vi "Data Viewer.vi"(8 "error in":errorcluster) -> (0 "error out":errorcluster)   [LabVIEW 2019, in "Report Viewer.lvlib" / "Report Viewer.lvclass"]
uses:
  Library/Report Viewer.lvclass
  Library/Report Viewer.lvclass/Report Viewer.ctl
  Accessors/Write Filename_ref.vi
  Accessors/GUI/Write Tree Refnum.vi
  Accessors/GUI/Write Graph_Ref.vi
  Accessors/GUI/Write Properties_Ref.vi
  Accessors/GUI/Write Values_Ref.vi
  Accessors/GUI/Write VI Refnum.vi
  Accessors/GUI/Write Save Data Button.vi
  Private/Tree/Clear Tree.vi
panel:
  in  "File contents":string[](tree)
  in  "Stop":bool
  out "File Name":string
  in  "Settings":bool
  in  "Open TDMS":bool
  in  "Save Graph":bool
  in  "Export Table":bool
  in  "Tab Control":T1(tab)
  in  "Properties Table":i32(listbox)
  in  "Values Table":i32(listbox)
  out "Waveform Graph":waveform(dbl)[](graph)
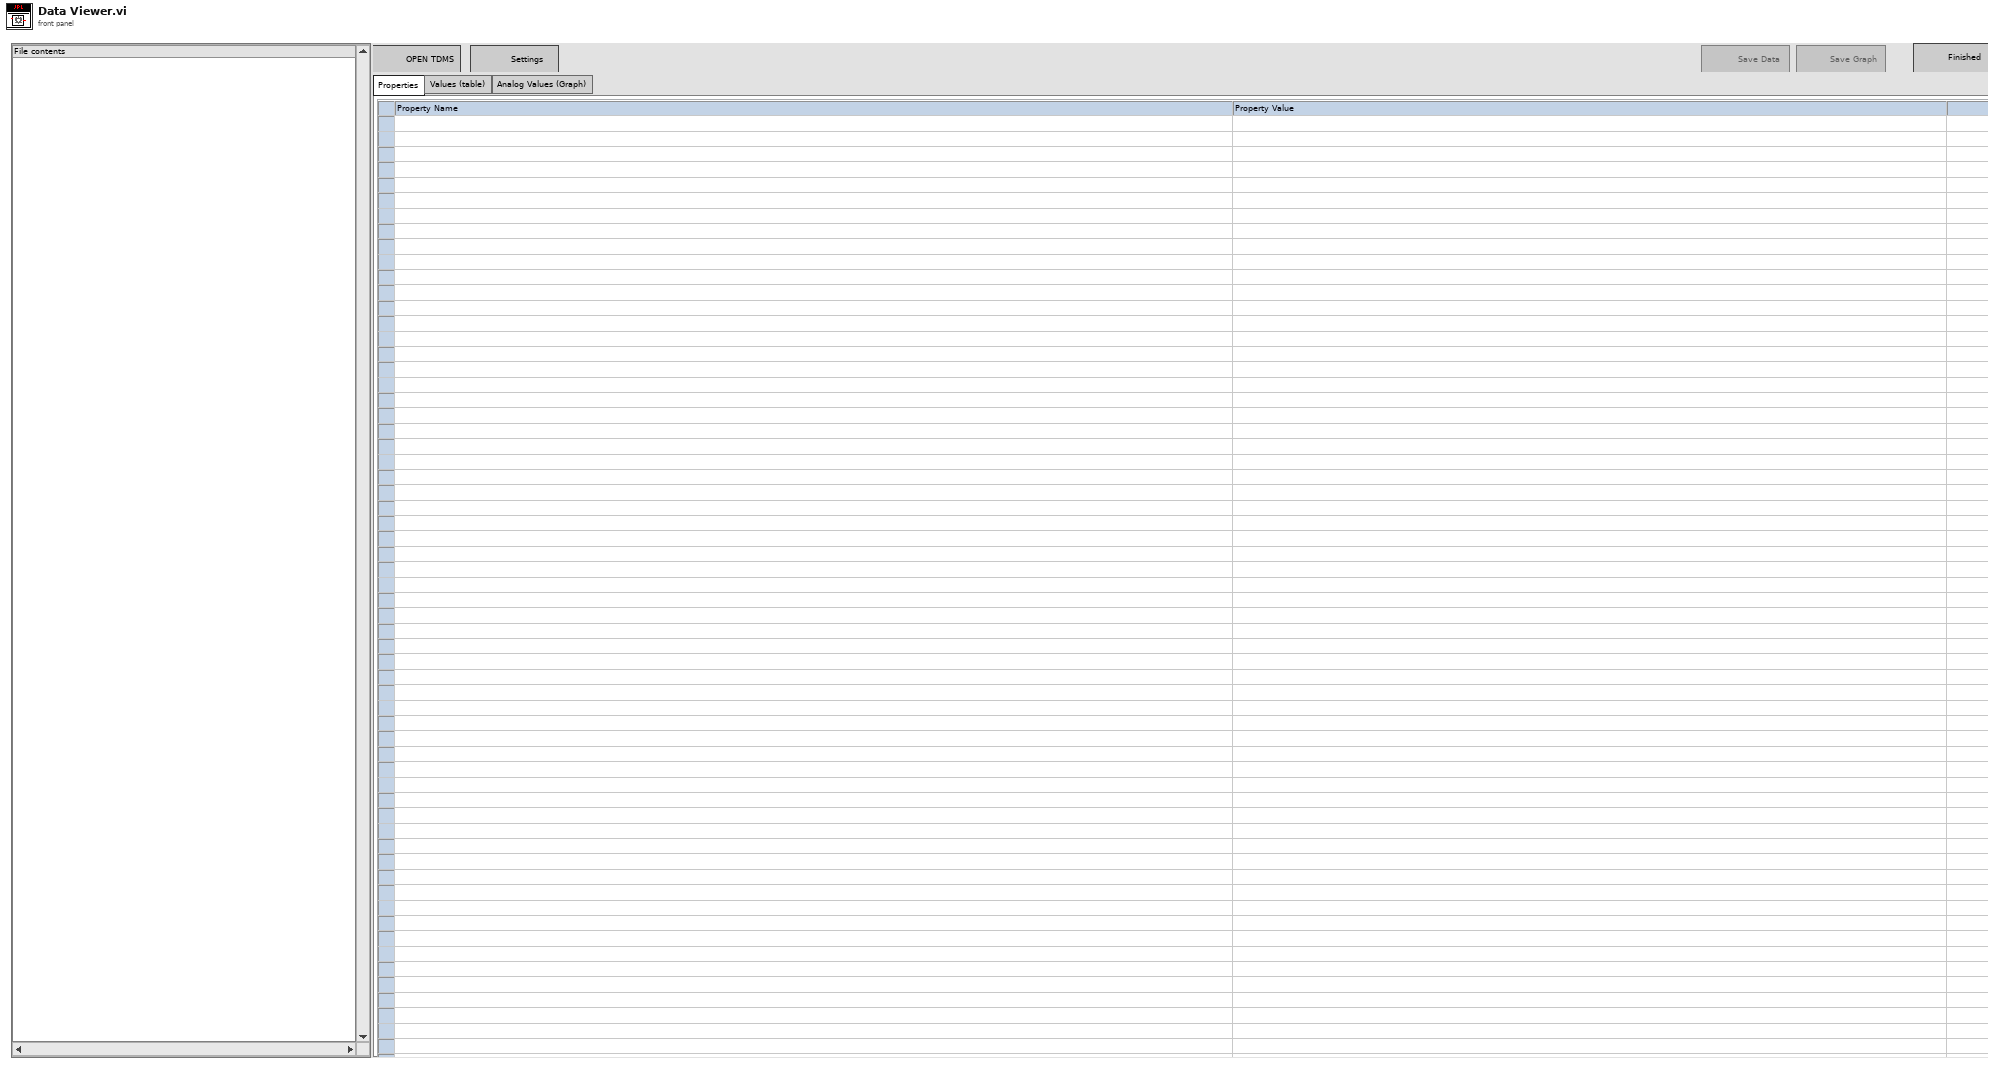
[diagram p1: front panel]
types:
  T1 = enum32{"Properties", "Values (table)", "Analog Values (Graph)"}
  T2 = typedef "LVBoundsTypeDef.ctl" = cluster{"Width":u32, "Height":u32}
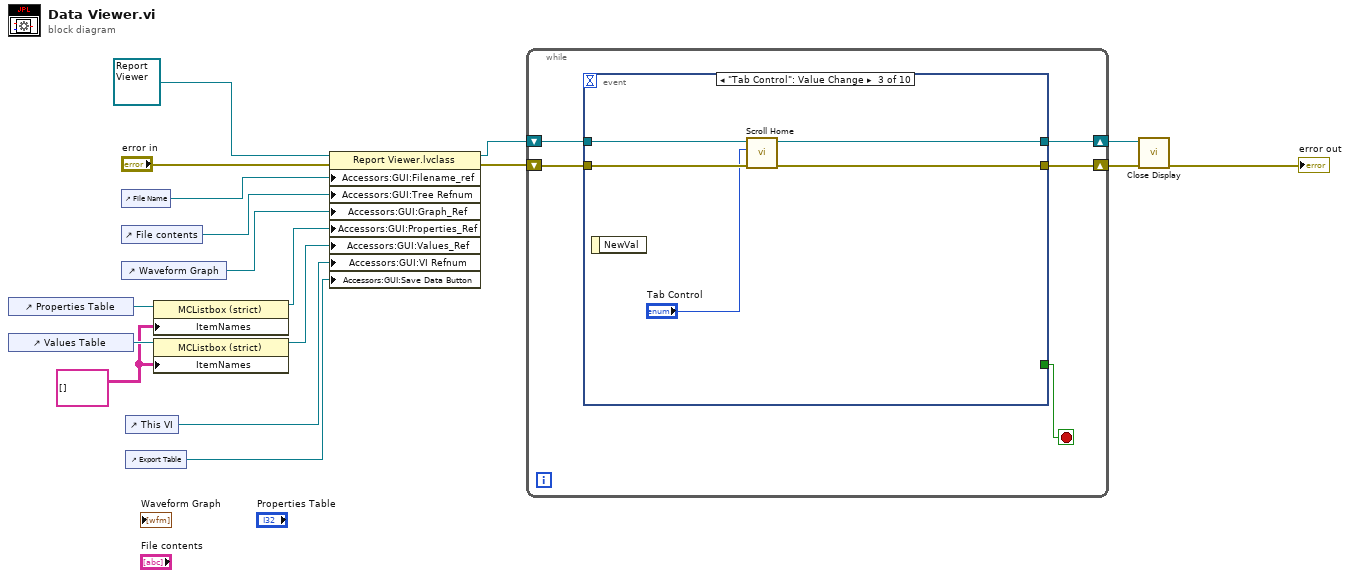
[diagram p0: block diagram]
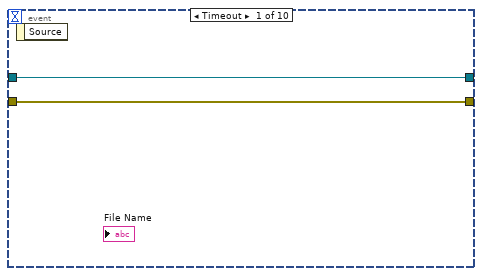
[diagram p2: hidden frame]
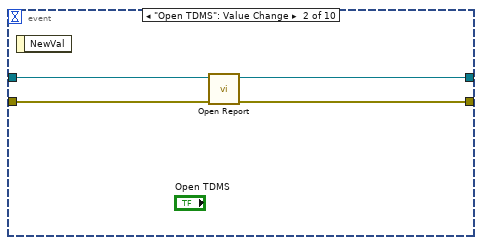
[diagram p3: hidden frame]
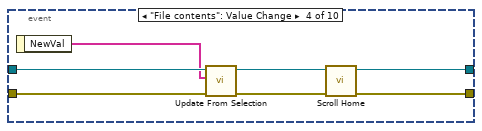
[diagram p4: hidden frame]
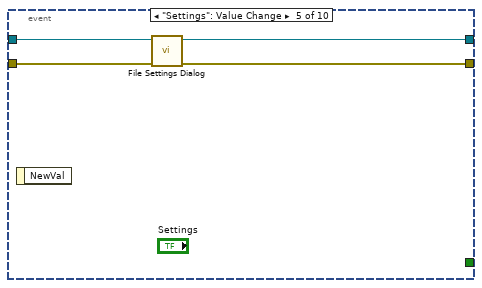
[diagram p5: hidden frame]
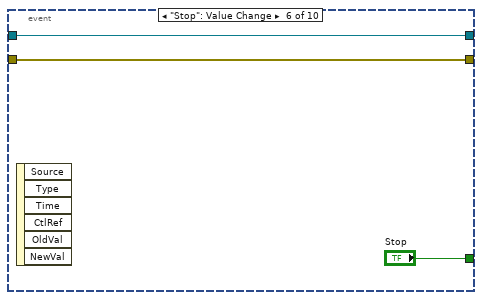
[diagram p6: hidden frame]
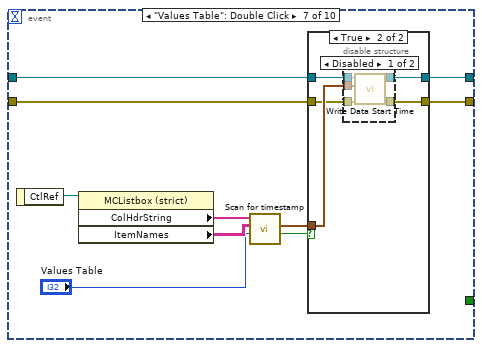
[diagram p7: hidden frame]
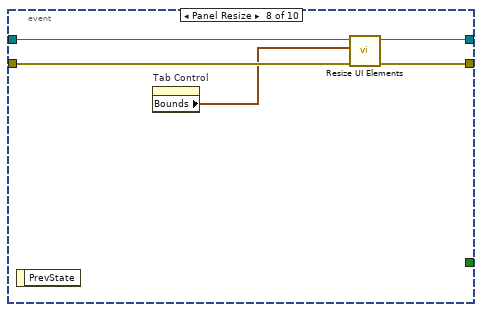
[diagram p10: hidden frame]
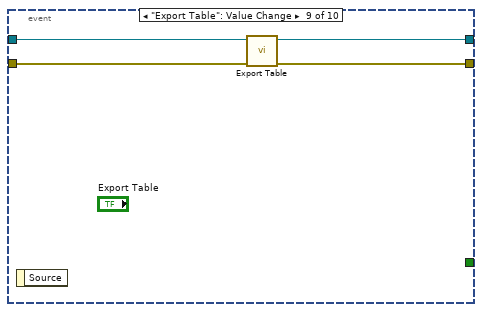
[diagram p11: hidden frame]
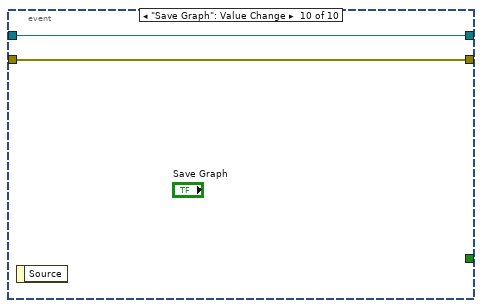
[diagram p12: hidden frame]
diagram:
  w5 = string[][] [] ("Item Names")
  n1 = control-ref of="Properties Table"() -> (w9:refnum<vi>)
  n2 = control-ref of="Values Table"() -> (w7:refnum<vi>)
  n3 = control-ref of="File Name"() -> (w14:refnum<vi>)
  n4 = control-ref of="File contents"() -> (w13:refnum<vi>)
  n5 = control-ref of="Waveform Graph"() -> (w12:refnum<vi>)
  n6 = control-ref of="This VI"() -> (w10:refnum<vi>)
  n7 = control-ref of="Export Table"() -> (w1:refnum<vi>)
  n8 = property class="MCListbox (strict)"(reference=w9, "ItemNames"=w5) -> (reference out=w8:refnum<vi>)  [unwired: 1 in, 1 out]
  n9 = property class="MCListbox (strict)"(reference=w7, "ItemNames"=w5) -> (reference out=w6:refnum<vi>)  [unwired: 1 in, 1 out]
  n10 = property class="Report Viewer.lvclass"(reference=refnum<class "Report Viewer.lvclass"> refnum ("Report Viewer in"), error in="error in", "Accessors:GUI:Filename_ref"=w14, "Accessors:GUI:Tree Refnum"=w13, "Accessors:GUI:Graph_Ref"=w12, "Accessors:GUI:Properties_Ref"=w8, "Accessors:GUI:Values_Ref"=w6, "Accessors:GUI:VI Refnum"=w10, "Accessors:GUI:Save Data Button"=w1) -> (reference out=w17:refnum<class "Report Viewer.lvclass">, error out=w11:errorcluster)
  n11 = while {
    shift-right: [w21] -> w3
    shift-left: w17 -> [w22]
    shift-right: [w18] -> w4
    shift-left: w11 -> [w20]
    stop <- w19 stop-if-true
    n12 = event shown="[2] \"Tab Control\": Value Change" {
      selector: _ -> [_ _ _ _ _ _ _ _ _ _]
      dyn-events: _ -> [_ _ _ _ _ _ _ _ _ _]
      timeout: _ -> [_ _ _ _ _ _ _ _ _ _]
      tunnel: w22 -> [w24 w28 w32 w40 w44 w46 w51 w76 w80 w82]
      tunnel: [w24 w27 w31 w35 w42 w46 w50 w74 w78 w82] -> w21
      tunnel: w20 -> [w23 w26 w33 w39 w43 w45 w48 w75 w79 w81]
      tunnel: [w23 w25 w30 w34 w41 w45 w49 w73 w77 w81] -> w18
      tunnel: [_ _ _ _ _ "Stop" _ _ _ _] -> w19
      event Timeout {
        n13 = event-data() -> ()  [unwired: 1 in, 1 out]
      }
      event "Open TDMS": Value Change {
        n14 = event-data() -> ()  [unwired: 1 in, 1 out]
        n15 = call "Open Report.vi"("error in"=w26, "Report Viewer in"=w28) -> ("error out"=w25:errorcluster, "Report Viewer out"=w27:refnum<class "Report Viewer.lvclass">)  [unwired: 8 in]
      }
      event "Tab Control": Value Change {
        n16 = event-data() -> ()  [unwired: 1 in, 1 out]
        n17 = call "Scroll Home.vi"("error in"=w33, "Tab Control"="Tab Control", "Report Viewer in"=w32) -> ("error out"=w30:errorcluster, "Report Viewer out"=w31:refnum<class "Report Viewer.lvclass">)  [unwired: 7 in]
      }
      event "File contents": Value Change {
        n18 = event-data() -> ("NewVal"=w38:string[])  [unwired: 1 in]
        n19 = call "Update From Selection.vi"("error in"=w39, "File Contents"=w38, "Report Viewer in"=w40) -> ("error out"=w36:errorcluster, "Report Viewer out"=w37:refnum<class "Report Viewer.lvclass">)  [unwired: 7 in]
        n20 = call "Scroll Home.vi"("error in"=w36, "Report Viewer in"=w37) -> ("error out"=w34:errorcluster, "Report Viewer out"=w35:refnum<class "Report Viewer.lvclass">)  [unwired: 8 in]
      }
      event "Settings": Value Change {
        n21 = event-data() -> ()  [unwired: 1 in, 1 out]
        n22 = call "File Settings Dialog.vi"("error in"=w43, "Report Viewer in"=w44) -> ("error out"=w41:errorcluster, "Report Viewer out"=w42:refnum<class "Report Viewer.lvclass">)  [unwired: 8 in]
      }
      event "Stop": Value Change {
        n23 = event-data() -> ()  [unwired: 1 in, 6 out]
      }
      event "Values Table": Double Click {
        n24 = event-data() -> ("CtlRef"=w57:refnum<vi>)  [unwired: 1 in]
        n25 = property class="MCListbox (strict)"(reference=w57) -> ("ColHdrString"=w56:string[], "ItemNames"=w55:string[][])  [unwired: 1 in, 2 out]
        n26 = call "Scan for timestamp.vi"("Row Index"="Values Table", "Item Names"=w55, "Column Headers"=w56) -> ("found"=w53:bool, "Time Stamp"=w52:timestamp)  [unwired: 7 in]
        n27 = case shown="True" w53 {
          tunnel: w52 -> [_ w63]
          tunnel: w51 -> [w59 w64]
          tunnel: [w59 w62] -> w50
          tunnel: [w58 w61] -> w49
          tunnel: w48 -> [w58 w60]
          frame False {
          }
          frame True {
            n28 = disable-structure shown="Disabled" {
              disable-tunnel: w64 -> [w69 w71]
              disable-tunnel: w63 -> [w68 _]
              disable-tunnel: [w67 w71] -> w62
              disable-tunnel: [w66 w70] -> w61
              disable-tunnel: w60 -> [w65 w70]
              frame Disabled {
                n29 = call "Write Data Start Time.vi"("error in"=w65, "Data Start Time"=w68, "Report Viewer in"=w69) -> ("error out"=w66:errorcluster, "Report Viewer out"=w67:refnum<class "Report Viewer.lvclass">)  [unwired: 7 in]
              }
              frame Enabled {
              }
            }
          }
        }
      }
      event Panel Resize {
        n30 = event-data() -> ()  [unwired: 1 in, 1 out]
        n31 = property on="Tab Control" class="TabCtl (strict)"() -> ("Bounds"=w72:T2)  [unwired: 2 in, 2 out]
        n32 = call "Resize UI Elements.vi"("error in (no error)"=w75, "New Tab dimensions"=w72, "Report Viewer in"=w76) -> ("error out"=w73:errorcluster, "Report Viewer out"=w74:refnum<class "Report Viewer.lvclass">)  [unwired: 7 in]
      }
      event "Export Table": Value Change {
        n33 = event-data() -> ()  [unwired: 1 in, 1 out]
        n34 = call "Export Table.vi"("error in (no error)"=w79, "Report Viewer in"=w80) -> ("error out"=w77:errorcluster, "Report Viewer out"=w78:refnum<class "Report Viewer.lvclass">)  [unwired: 8 in]
      }
      event "Save Graph": Value Change {
        n35 = event-data() -> ()  [unwired: 1 in, 1 out]
      }
    }
  }
  n36 = call "Close Display.vi"("error in (no error)"=w4, "Report Viewer in"=w3) -> ("error out"=→"error out":errorcluster)  [unwired: 8 in, 1 out]
